vi "Profit Over Time.vi"() -> ()   [LabVIEW 2021]
panel:
  out "residual":dbl
  out "Top 5 Profiteers":T1(array[cluster])
  out "Profits during time period":T2(array[cluster])
  out "End Date":timestamp format="%<%x>T"
  out "Start Date":timestamp format="%<%x>T"
  in  "file path (use dialog)":path=path "C:/Users/manma/Google Drive/WPC Stat Scrape/Data/WPC Stats.bin"
  in  "# of updates back":u16=15
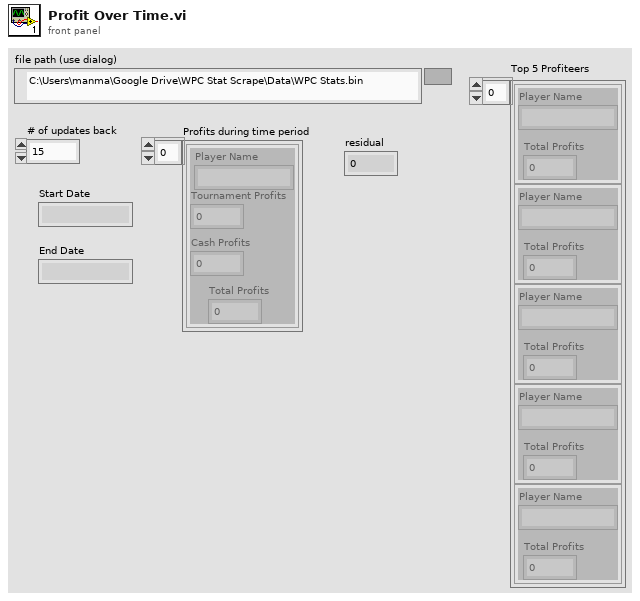
[diagram p1: front panel]
types:
  T1 = cluster{"Player Name":string, "Total Profits":dbl}[]
  T2 = cluster{"Player Name":string, "Tournament Profits":dbl, "Cash Profits":dbl, "Total Profits":dbl}[]
  T3 = typedef "WPC Player and Financial Stats.ctl" = cluster{"Player Name":string, "Date Updated":timestamp, "Tournament Stats":cluster{"Hands Won":i32, "Hands Played":i32, "Hands Dealt":i32, "All-Ins":i32, "Entered":i32, "Winnings":dbl, "Profit":dbl}, "Cash Stats":cluster{"Hands Won":i32, "Hands Played":i32, "Hands Dealt":i32, "All-Ins":i32, "Profit":dbl}}
  T4 = cluster{"Hands Won":i32, "Hands Played":i32, "Hands Dealt":i32, "All-Ins":i32, "Entered":i32, "Winnings":dbl, "Profit":dbl}
  T5 = cluster{"Hands Won":i32, "Hands Played":i32, "Hands Dealt":i32, "All-Ins":i32, "Profit":dbl}
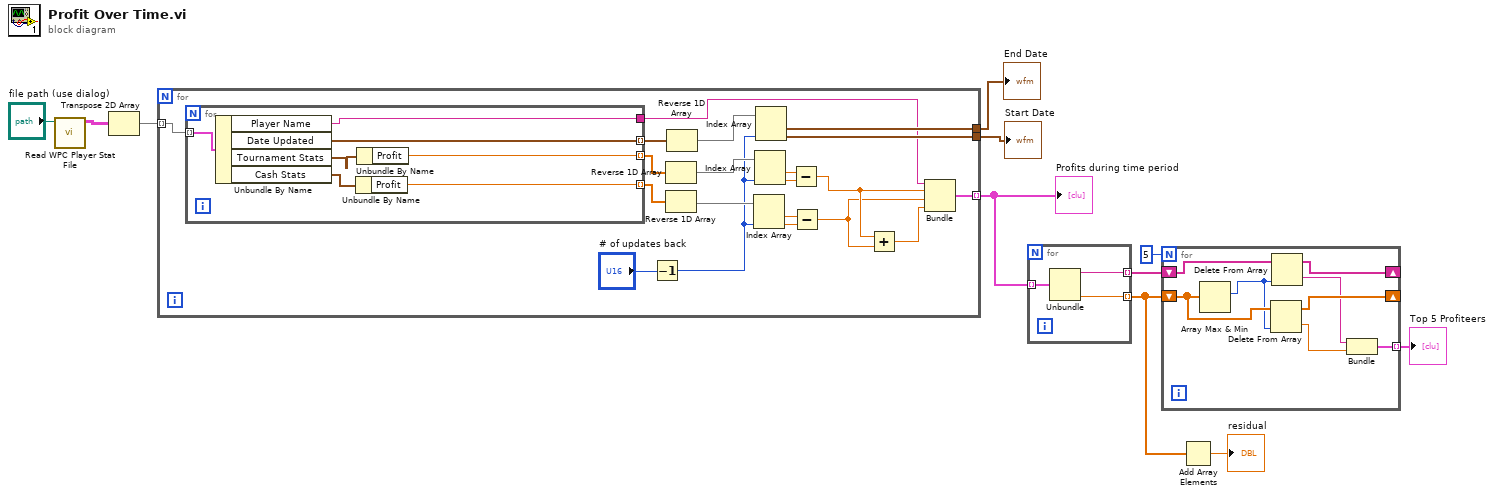
[diagram p0: block diagram]
diagram:
  n1 = call "Read WPC Player Stat File.vi"("file path (use dialog)"="file path (use dialog)") -> ("Full WPC Stats"=w10:T3[][])  [unwired: 8 in, 2 out]
  n2 = Transpose 2D Array(2D array=w10) -> (transposed array=w11:T3[][])
  n3 = for {
    tunnel: w11 -> [w31] mode=indexing
    tunnel: [w22] -> w7
    tunnel: [w21] -> w8
    tunnel: [w12] -> w6 mode=indexing
    n4 = for {
      tunnel: w31 -> [w38] mode=indexing
      tunnel: [w37] -> w16
      tunnel: [w36] -> w30 mode=indexing
      tunnel: [w33] -> w29 mode=indexing
      tunnel: [w32] -> w28 mode=indexing
      n5 = Unbundle By Name(w38) -> ("Player Name"=w37:string, "Date Updated"=w36:timestamp, "Tournament Stats"=w35:T4, "Cash Stats"=w34:T5)
      n6 = Unbundle By Name(w34) -> ("Profit"=w32:dbl)
      n7 = Unbundle By Name(w35) -> ("Profit"=w33:dbl)
    }
    n8 = Decrement(x="# of updates back") -> (x-1=w23:u16)
    n9 = Reverse 1D Array(array=w29) -> (reversed array=w26:dbl[])
    n10 = Reverse 1D Array(array=w28) -> (reversed array=w25:dbl[])
    n11 = Reverse 1D Array(array=w30) -> (reversed array=w27:timestamp[])
    n12 = Index Array(array=w25, index #2=w23) -> (element #1=w18:dbl, element #2=w17:dbl)  [unwired: 1 in]
    n13 = Index Array(array=w26, index #2=w23) -> (element #1=w19:dbl, element #2=w20:dbl)  [unwired: 1 in]
    n14 = Index Array(array=w27, index #2=w23) -> (element #1=w22:timestamp, element #2=w21:timestamp)  [unwired: 1 in]
    n15 = Subtract(x=w19, y=w20) -> (x-y=w15:dbl)
    n16 = Subtract(x=w18, y=w17) -> (x-y=w14:dbl)
    n17 = Add(x=w15, y=w14) -> (x+y=w13:dbl)
    n18 = Bundle("Player Name"=w16, w15, w14, w13) -> (w12:cluster{"Player Name":string, dbl, dbl, dbl})  [unwired: 1 in]
  }
  "Start Date" <- w8
  "End Date" <- w7
  "Profits during time period" <- w6
  n19 = for {
    tunnel: w6 -> [w41] mode=indexing
    tunnel: [w40] -> w5 mode=indexing
    tunnel: [w39] -> w2 mode=indexing
    n20 = Unbundle(w41) -> ("Player Name"=w40:string, w39:dbl)  [unwired: 2 out]
  }
  n21 = for {
    N: 5 -> [_]
    shift-right: [w45] -> _
    shift-left: w2 -> [w49]
    shift-right: [w46] -> _
    shift-left: w5 -> [w48]
    tunnel: [w42] -> w3 mode=indexing
    n22 = Array Max & Min(array=w49) -> (max index (indices)=w47:i32)  [unwired: 3 out]
    n23 = Delete From Array(array=w49, index=w47) -> (deleted portion=w43:dbl, array with subset deleted=w45:dbl[])  [unwired: 1 in]
    n24 = Delete From Array(array=w48, index=w47) -> (deleted portion=w44:string, array with subset deleted=w46:string[])  [unwired: 1 in]
    n25 = Bundle("Player Name"=w44, w43) -> (w42:cluster{"Player Name":string, dbl})  [unwired: 1 in]
  }
  "Top 5 Profiteers" <- w3
  n26 = Add Array Elements(numeric array=w2) -> (sum=→"residual":dbl)
